vi "Read LNA Status.vi"(8 "error in (no error)":errorcluster, 11 "CS++RTMainActor in":refnum<class "CS++RTMainActor.lvclass">) -> (0 "error out":errorcluster, 2 "LNA Status":T1, 3 "CS++RTMainActor out":refnum<class "CS++RTMainActor.lvclass">)   [LabVIEW 2016, in "CS++RTMain.lvlib" / "CS++RTMainActor.lvclass"]
uses:
  CS++RTMainActor.lvclass
  CS++RTMainActor.lvclass/CS++RTMainActor.ctl
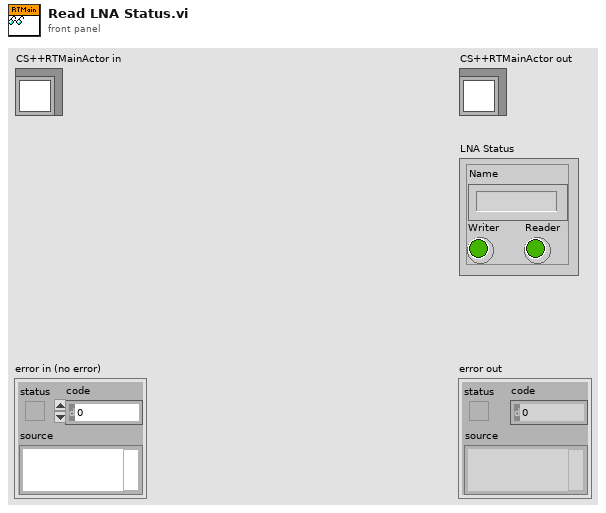
[diagram p1: front panel]
types:
  T1 = cluster{"Name":string, "Writer":bool, "Reader":bool}
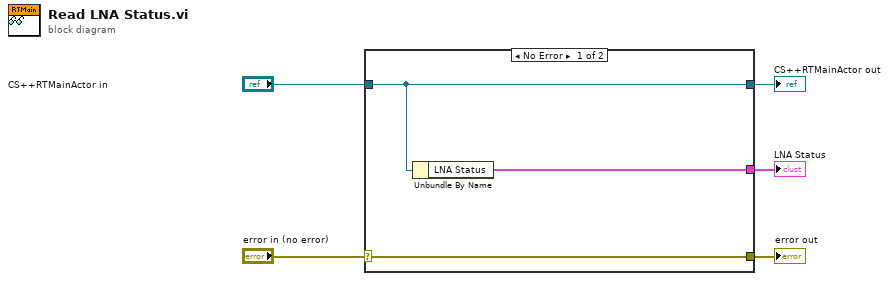
[diagram p0: block diagram]
diagram:
  n1 = case shown="No Error" "error in (no error)" {
    selector: "error in (no error)" -> [w8 w9]
    tunnel: [w8 w9] -> w4
    tunnel: [w7 w10] -> w2
    tunnel: "CS++RTMainActor in" -> [w7 w10]
    tunnel: [w6 _] -> w1
    frame No Error {
      n2 = Unbundle By Name(w7) -> ("LNA Status"=w6:T1)
    }
    frame Error {
    }
  }
  "error out" <- w4
  "CS++RTMainActor out" <- w2
  "LNA Status" <- w1
